vi "PCO_GetBinning.vi"(8 "error in (no error)":errorcluster {"code" format="%x"}, 11 "ph":u64) -> (0 "error out":errorcluster {"code" format="%x"}, 1 "wBinHorz":u16, 2 "ErrorMessage":i32 format="%x", 3 "ph out":u64, 5 "wBinVert":u16)   [LabVIEW 2019, in "SDK.lvlib" / "ImageSensor.lvlib"]
doc: "<b>Description:</b>\nThis function returns the current binning setting of the camera values for horizontal and vertical direction.\n\n<b>Supported camera type:</b>\nAll cameras\n\n<b>Descriptor dependency:</b>\nNone"
uses:
  ImageSensor.lvlib
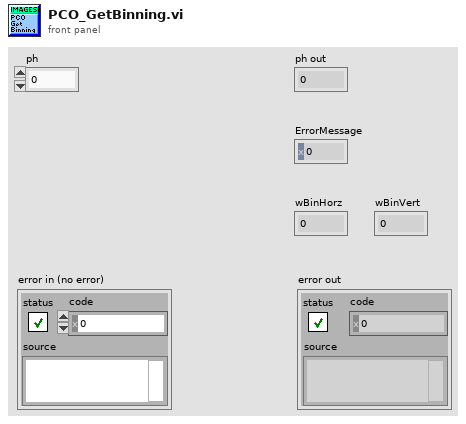
[diagram p1: front panel]
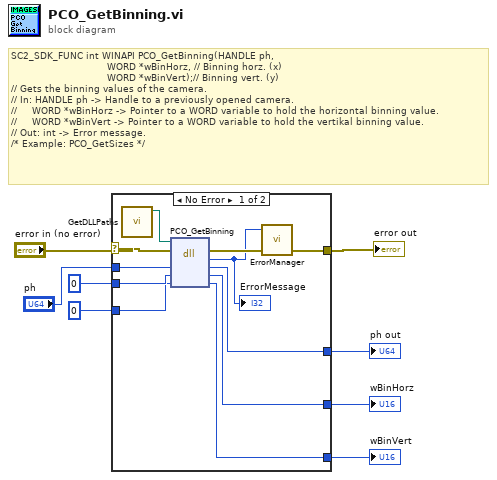
[diagram p0: block diagram]
diagram:
  # "SC2_SDK_FUNC int WINAPI PCO_GetBinning(HANDLE ph,\n                                WORD *wBinHorz, // Binning horz. (x)\n                                WORD *wBinVert);// Binning vert. (y)\n// Gets the binning values of the camera.\n// In: HANDLE ph -> Handle to a previously opened camera.\n//     WORD *wBinHorz -> Pointer to a WORD variable to hold the horizontal binning value.\n//     WORD *wBinVert -> Pointer to a WORD variable to hold the vertikal binning value.\n// Out: int -> Error message.\n/* Example: PCO_GetSizes */"
  n1 = case shown="No Error" "error in (no error)" {
    selector: "error in (no error)" -> [w10 w23]
    tunnel: "ph" -> [w19 w22]
    tunnel: u16 0 ("wBinHorz") -> [w18 w21]
    tunnel: [w17 w21] -> w6
    tunnel: u16 0 ("wBinVert") -> [w16 w20]
    tunnel: [w15 w20] -> w4
    tunnel: [w14 w22] -> w3
    tunnel: [w12 w23] -> w2
    frame No Error {
      n2 = call "GetDLLPaths.vi"() -> ("SC2_Cam_Path"=w9:path)  [unwired: 9 in, 2 out]
      n3 = dll-call lib="?" fn="PCO_GetBinning"(path in=w9, error in=w10, "ph"=w19, "wBinHorz"=w18, "wBinVert"=w16) -> (error out=w13:errorcluster, "return type"=w11:i32, "ph"=w14:u64, "wBinHorz"=w17:u16, "wBinVert"=w15:u16)  [unwired: 1 in, 1 out]
      "ErrorMessage" <- w11
      n4 = call "ErrorManager.vi"("error in (no error)"=w13, "error code"=w11) -> ("error out"=w12:errorcluster)  [unwired: 3 in]
    }
    frame Error {
    }
  }
  "ph out" <- w3
  "wBinHorz" <- w6
  "wBinVert" <- w4
  "error out" <- w2
